vi "Lab1_2.vi"() -> ()   [LabVIEW 2020]
panel:
  in  "Start Button":bool
  out "Array":i32[](array[numeric])
  in  "stop":bool
  out "x+y":i32
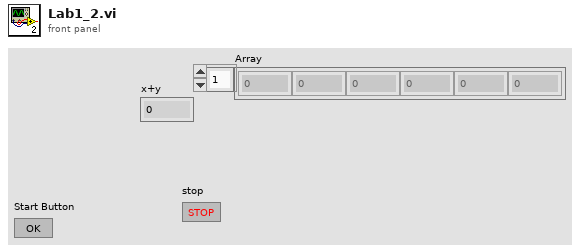
[diagram p1: front panel]
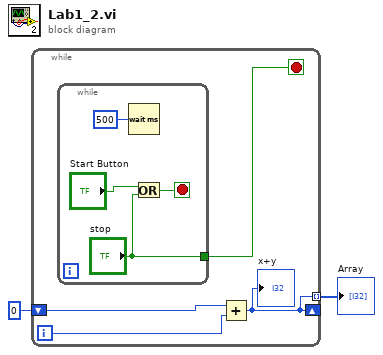
[diagram p0: block diagram]
diagram:
  n1 = while {
    shift-right: [w3] -> _
    shift-left: 0 -> [w5]
    tunnel: [w3] -> w1 mode=indexing
    i -> [w6]
    stop <- w4 stop-if-true
    n2 = while {
      tunnel: ["stop"] -> w4
      stop <- w10 stop-if-true
      n3 = Wait (ms)(milliseconds to wait=u32 500) -> ()  [unwired: 1 out]
      n4 = Or(x="Start Button", y="stop") -> (x .or. y?=w10:bool)
    }
    n5 = Add(x=w5, y=w6) -> (x+y=w3:i32)
    "x+y" <- w3
  }
  "Array" <- w1
